vi "local file settings to globals.vi"(8 "error in (no error)":errorcluster, 10 "FPGA HW Detected":bool, 11 "DAQ FPGA Settings":T4) -> (0 "error out":errorcluster, 3 "DAQ FPGA Settings":T3)   [LabVIEW 2020]
uses:
  TypeDef/FPGA_DAQ_settings.ctl
  TypeDef/FPGA_adapter_type.ctl
  TypeDef/FPGA_card_type.ctl
  Globals/FPGA Globals.vi
panel:
  out "Adapter Module":T1
  out "FPGA Card":T2
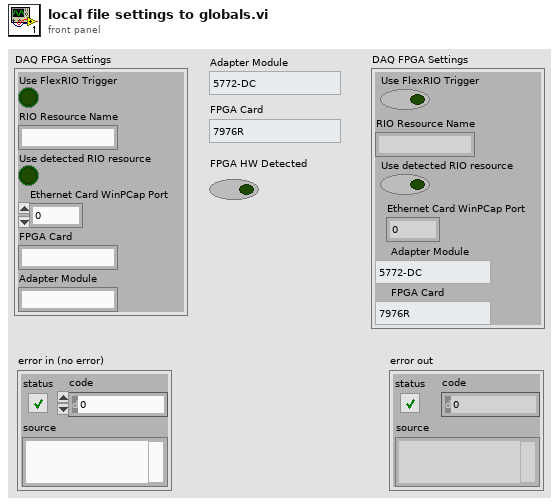
[diagram p1: front panel]
types:
  T1 = typedef "FPGA_adapter_type.ctl" = enum16{"5772-DC", "5772-AC"}
  T2 = typedef "FPGA_card_type.ctl" = enum16{"7976R", "7975R", "7966R"}
  T3 = typedef "FPGA_DAQ_settings.ctl" = cluster{"Use FlexRIO Trigger":bool, "RIO Resource Name":string, "Use detected RIO resource":bool, "Ethernet Card WinPCap Port ":i16, "Adapter Module":T1, "FPGA Card":T2}
  T4 = cluster{"Use FlexRIO Trigger":bool, "RIO Resource Name":string, "Use detected RIO resource":bool, "Ethernet Card WinPCap Port ":i16, "FPGA Card":string, "Adapter Module":string}
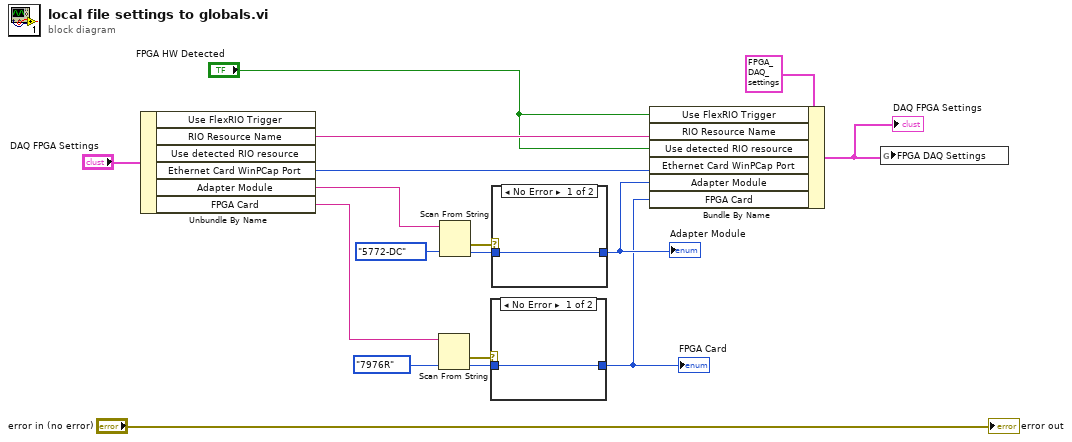
[diagram p0: block diagram]
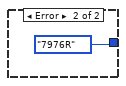
[diagram p2: hidden frame]
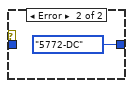
[diagram p3: hidden frame]
diagram:
  n1 = Unbundle By Name("DAQ FPGA Settings") -> ("RIO Resource Name"=w14:string, "Ethernet Card WinPCap Port"=w13:i16, "Adapter Module"=w9:string, "FPGA Card"=w4:string)  [unwired: 2 out]
  n2 = Scan From String(input string=w4, default 1=FPGA_card_type."7976R" ("FPGA Card")) -> (error out=w5:errorcluster, output 1=w6:T2)  [unwired: 3 in, 2 out]
  n3 = Scan From String(input string=w9, default 1=FPGA_adapter_type."5772-DC" ("Adapter Module")) -> (error out=w11:errorcluster, output 1=w10:T1)  [unwired: 3 in, 2 out]
  n4 = case shown="No Error" w5 {
    tunnel: w6 -> [w18 _]
    tunnel: [w18 enum16{"7976R", "7975R"}."7976R" ("FPGA Card")] -> w2
    frame No Error {
    }
    frame Error {
    }
  }
  "FPGA Card" <- w2
  n5 = case shown="No Error" w11 {
    tunnel: w10 -> [w20 _]
    tunnel: [w20 enum16{"5772-DC", "5772-AC"}."5772-DC" ("Adapter Module")] -> w8
    frame No Error {
    }
    frame Error {
    }
  }
  "Adapter Module" <- w8
  n6 = Bundle By Name(cluster=T3 {"Use FlexRIO Trigger"=FALSE, "RIO Resource Name"="", "Use detected RIO resource"=FALSE, "Ethernet Card WinPCap Port "=0, "Adapter Module"=enum."5772-DC", "FPGA Card"=enum."7976R"} ("FPGA DAQ Settings"), "Use FlexRIO Trigger"="FPGA HW Detected", "RIO Resource Name"=w14, "Use detected RIO resource"="FPGA HW Detected", "Ethernet Card WinPCap Port"=w13, "Adapter Module"=w8, "FPGA Card"=w2) -> (w15:T3)
  "DAQ FPGA Settings" <- w15
  n7 = global write "FPGA Globals.vi" "FPGA DAQ Settings"(w15) -> ()
  "error out" <- "error in (no error)"
